vi "kinectRead [Infrared Frame].vi"(8 "Error In":errorcluster, 9 "Timeout (ms)":i32=5000, 11 "KinectSensor References in":T1) -> (0 "Error Out":errorcluster, 2 "frameData":dbl[](array[numeric]), 3 "KinectSensor References out":T1)   [LabVIEW 2011, in "KinectOne.lvlib"]
uses:
  KinectOne.lvlib
  Type Defs/KinectSensor References.ctl
  Microsoft.Kinect
  C:/github/makerhub/KinectOne/LabVIEW/vi.lib/MakerHub/KinectOne/Private/Libs/BodyFrameDataInterface.dll
  Libs/BodyFrameDataInterface.dll
  Frame Data FGV [Infrared].vi
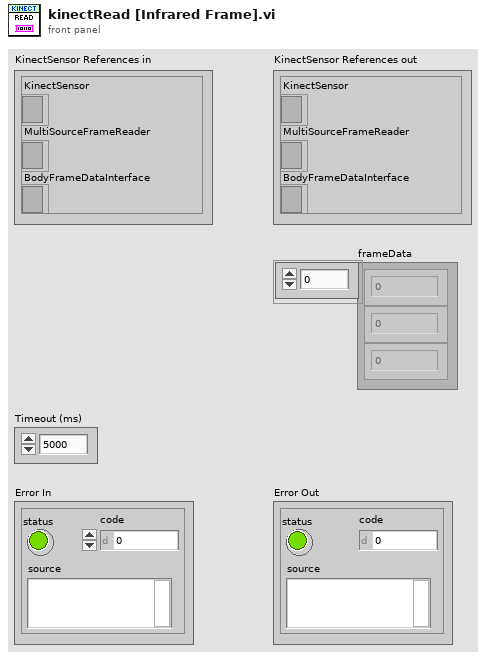
[diagram p1: front panel]
types:
  T1 = typedef "KinectOne.lvlib/KinectSensor References.ctl" = cluster{"KinectSensor":refnum<k24>, "MultiSourceFrameReader":refnum<k24>, "BodyFrameDataInterface":refnum<k24>}
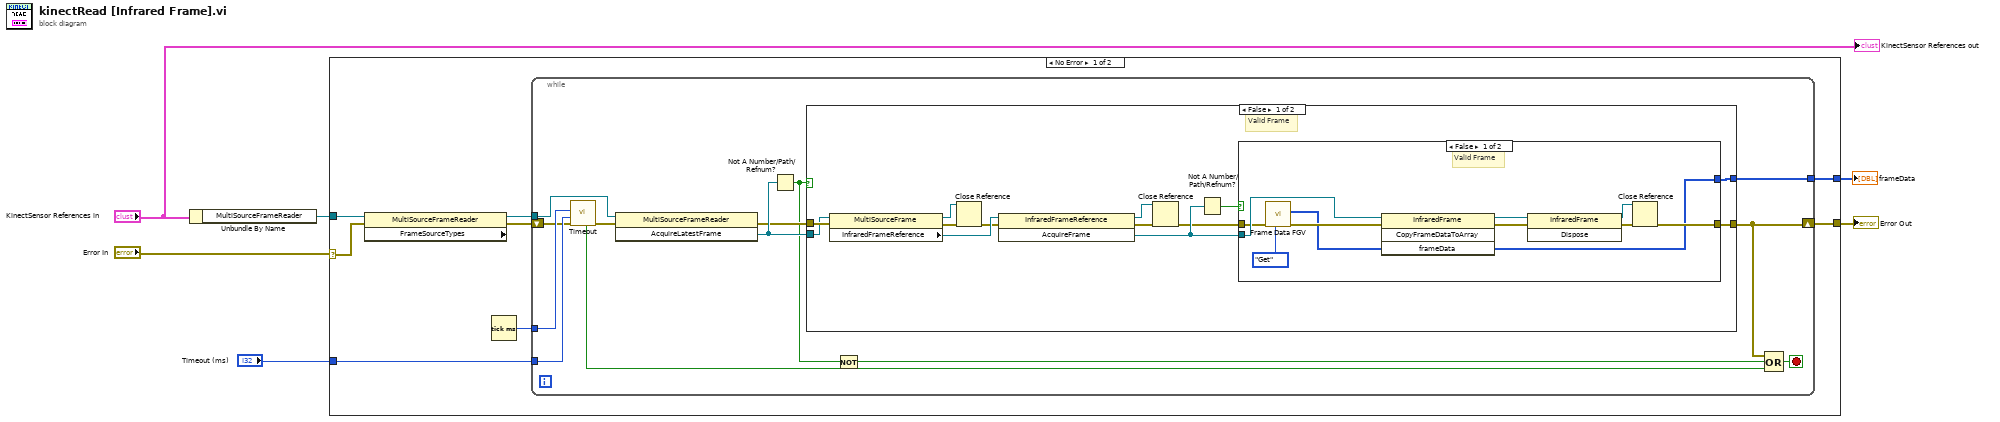
[diagram p0: block diagram]
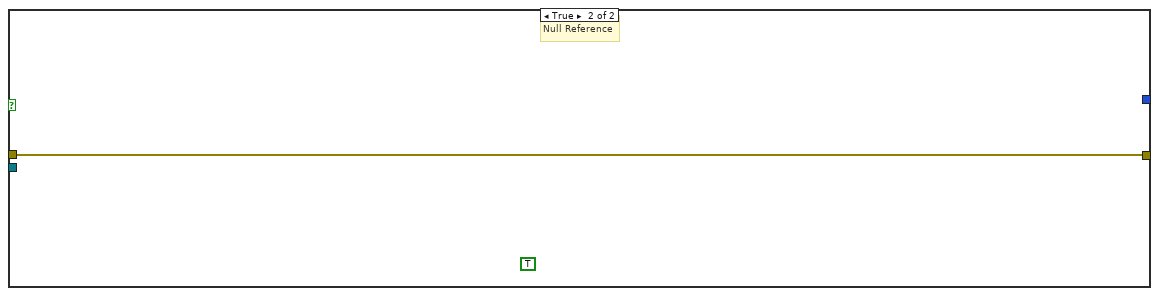
[diagram p3: hidden frame]
diagram:
  n1 = Unbundle By Name("KinectSensor References in") -> ("MultiSourceFrameReader"=w6:refnum<k24>)
  n2 = case shown="No Error" "Error In" {
    selector: "Error In" -> [w9 w54]
    tunnel: w6 -> [w12 _]
    tunnel: [w11 w54] -> w1
    tunnel: [w10 _] -> w4
    tunnel: "Timeout (ms)" -> [w7 _]
    frame No Error {
      n3 = property class="MultiSourceFrameReader" props=["FrameSourceTypes"](reference=w12, error in=w9) -> (reference out=w14:refnum<k24>, error out=w13:errorcluster)  [unwired: 1 out]
      n4 = Tick Count (ms)() -> (millisecond timer value=w8:u32)
      n5 = while {
        tunnel: w14 -> [w20]
        shift-right: [w18] -> w11
        shift-left: w13 -> [w22]
        tunnel: [w25] -> w10
        tunnel: w8 -> [w24]
        tunnel: w7 -> [w23]
        stop <- w17 stop-if-true
        n6 = call "Timeout.vi"("error in (no error)"=w22, "Timeout (ms)"=w23, "Start Time"=w24) -> ("error out"=w21:errorcluster, "Timeout?"=w19:bool)  [unwired: 7 in]
        n7 = invoke class="MultiSourceFrameReader" method="AcquireLatestFrame"(reference=w20, error in=w21) -> (error out=w26:errorcluster, "AcquireLatestFrame"=w27:refnum<k24>)  [unwired: 1 in, 1 out]
        n8 = Not A Number/Path/Refnum?(number/path/refnum=w27) -> (NaN/Path/Refnum?=w16:bool)
        n9 = case shown="False" w16 {
          tunnel: w26 -> [w39 w53]
          tunnel: w27 -> [w36 _]
          tunnel: [w38 w53] -> w18
          tunnel: [w34 _] -> w25
          frame False {
            # "Valid Frame"
            n10 = property class="MultiSourceFrame"(reference=w36, error in=w39) -> (reference out=w32:refnum<k24>, error out=w33:errorcluster, "InfraredFrameReference"=w35:refnum<k24>)
            n11 = Close Reference(reference=w32, error in (no error)=w33) -> (error out=w31:errorcluster)
            n12 = invoke class="InfraredFrameReference" method="AcquireFrame"(reference=w35, error in=w31) -> (reference out=w29:refnum<k24>, error out=w30:errorcluster, "AcquireFrame"=w40:refnum<k24>)  [unwired: 1 in]
            n13 = Close Reference(reference=w29, error in (no error)=w30) -> (error out=w28:errorcluster)
            n14 = Not A Number/Path/Refnum?(number/path/refnum=w40) -> (NaN/Path/Refnum?=w37:bool)
            n15 = case shown="False" w37 {
              tunnel: w28 -> [w44 w52]
              tunnel: w40 -> [w47 _]
              tunnel: [w46 w52] -> w38
              tunnel: [w45 _] -> w34
              frame False {
                # "Valid Frame"
                n16 = call-poly "Frame Data FGV.vi"("Command"=enum16{"Get", "Initialize"}."Get", "error in (no error)"=w44) -> ("error out"=w43:errorcluster, "Array"=w42:u16[])  [unwired: 8 in]
                n17 = invoke class="InfraredFrame" method="CopyFrameDataToArray"(reference=w47, error in=w43, "frameData"=w42) -> (reference out=w48:refnum<k24>, error out=w49:errorcluster, "frameData"=w45:u16[])  [unwired: 1 in, 1 out]
                n18 = invoke class="InfraredFrame" method="Dispose"(reference=w48, error in=w49) -> (reference out=w51:refnum<k24>, error out=w50:errorcluster)  [unwired: 1 in, 1 out]
                n19 = Close Reference(reference=w51, error in (no error)=w50) -> (error out=w46:errorcluster)
              }
              frame True {
                # "Null Reference"
              }
            }
          }
          frame True {
            (unwired) TRUE
            # "Null Reference"
          }
        }
        n20 = Not(x=w16) -> (.not. x?=w15:bool)
        n21 = Compound Arithmetic op=OR(w18, w15, w19) -> (w17:bool)
      }
    }
    frame Error {
      # "Pass out upstream error"
    }
  }
  "Error Out" <- w1
  "frameData" <- w4
  "KinectSensor References out" <- "KinectSensor References in"
